vi "ws Auth Get-Set Kill.vi"(8 "error in (no error)":errorcluster, 11 "KillCode to Set (empty - read existing)":string) -> (0 "error out":errorcluster, 3 "KillCode":string)   [LabVIEW 2011]
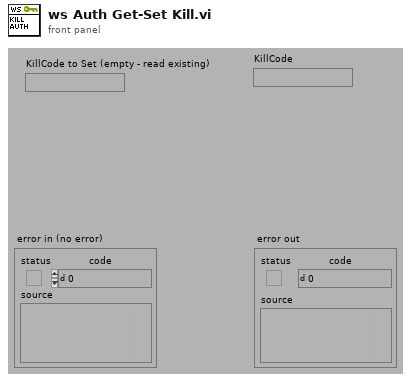
[diagram p1: front panel]
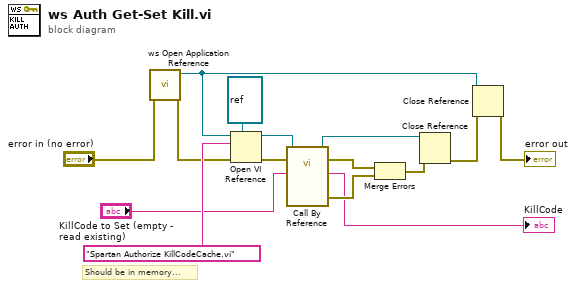
[diagram p0: block diagram]
diagram:
  # "Should be in memory..."
  n1 = call "ws Open Application Reference.vi"("error in (no error)"="error in (no error)") -> ("error out"=w2:errorcluster, "application reference"=w4:refnum<vi>)  [unwired: 9 in]
  n2 = Open VI Reference(type specifier VI Refnum (for type only)=refnum<vi> refnum, application reference (local)=w4, vi path="Spartan Authorize KillCodeCache.vi", error in (no error)=w2) -> (vi reference=w10:refnum<vi>, error out=w11:errorcluster)  [unwired: 2 in]
  n3 = call-by-ref "?"(reference=w10, error in=w11, "KillCode in (empty - just read from cache)"="KillCode to Set (empty - read existing)") -> (reference out=w9:refnum<vi>, error out=w8:errorcluster, 0:"error out"=w7:errorcluster, "KillCode out"=→"KillCode":string)  [unwired: 5 in]
  n4 = Merge Errors(w8, w7) -> (w13:errorcluster)
  n5 = Close Reference(reference=w9, error in (no error)=w13) -> (error out=w15:errorcluster)
  n6 = Close Reference(reference=w4, error in (no error)=w15) -> (error out=→"error out":errorcluster)
